vi "Cleanup TCP Connection.vi"(8 "error in (no error)":errorcluster, 11 "TCP Client in":refnum<class "TCP Client.lvclass">) -> (0 "error out":errorcluster, 3 "TCP Client out":refnum<class "TCP Client.lvclass">)   [LabVIEW 2020, in "Stream-TCP.lvlib" / "TCP Client.lvclass"]
uses:
  TCP Client.lvclass
  TCP Client.lvclass/TCP Client.ctl
  TCP Stream/TCP Stream.lvclass
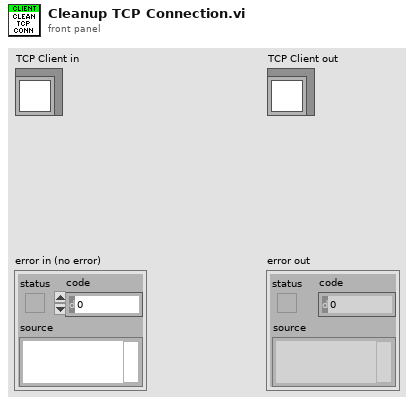
[diagram p1: front panel]
types:
  T1 = typedef "Stream-TCP.lvlib/TCP Client.lvclass/Ref Data.ctl" = cluster{"TCP Connection":refnum<k5>, "TCP Stream":refnum<class "TCP Stream.lvclass">, "State":T2, "Connection Loop":refnum<vi>}
  T2 = typedef "Stream-TCP.lvlib/TCP Client.lvclass/Connection State.ctl" = enum16{"Closed", "Idle", "Connecting", "Connected", "Shutdown"}
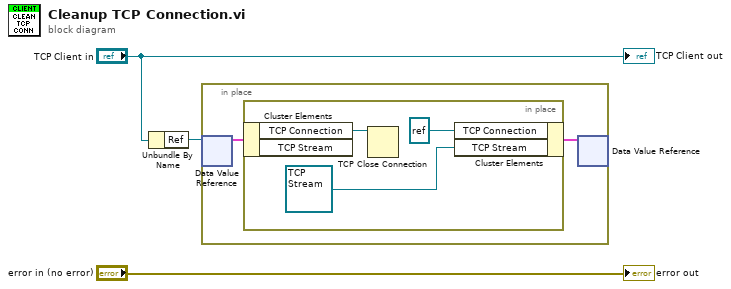
[diagram p0: block diagram]
diagram:
  n1 = Unbundle By Name("TCP Client in") -> ("Ref"=w2:refnum<data-value>)
  n2 = in-place {
    n3 = in-place-dvr #1(w2) -> (w5:T1)  [unwired: 1 out]
    n4 = in-place {
      n5 = in-place-cluster #2(w5) -> ("TCP Connection"=w7:refnum<k5>)  [unwired: 1 out]
      n6 = TCP Close Connection(connection ID=w7) -> ()  [unwired: 2 in, 2 out]
      n7 = in-place-cluster #2("TCP Connection"=refnum<k5> refnum, "TCP Stream"=refnum<class "TCP Stream.lvclass"> refnum) -> (w4:T1)
    }
    n8 = in-place-dvr #1(w4) -> ()  [unwired: 2 out]
  }
  "error out" <- "error in (no error)"
  "TCP Client out" <- "TCP Client in"
